vi "LoadCalcParPanel.vi"(4 "CalcProgQEvent":refnum<user-event>, 6 "CalcProgQ":refnum<queue>, 8 "error in (no error)":errorcluster caption="entrée d'erreur (pas d'erreur)", 9 "Session":i32, 11 "RemPanRef":refnum<vi>) -> (0 "sortie d'erreur":errorcluster, 2 "InstrClassEventQ":T1(array[cluster]), 3 "PanelViRefOut":refnum<vi>[](array[refnum]))   [LabVIEW 2019]
uses:
  Calculations Class/Calculations.lvclass
  C:/Programmes Labview/LabScanV1A/DevicesClass/BaseDevice/BaseDevice.lvclass
  DevicesClass/BaseDevice/BaseDevice.lvclass
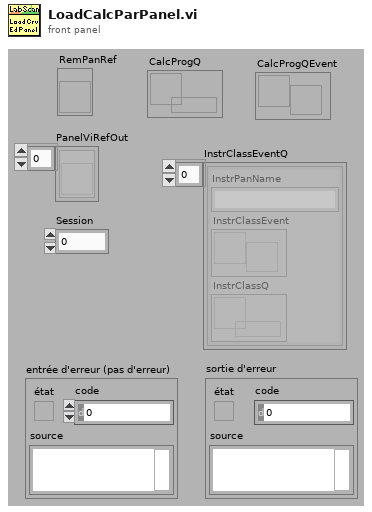
[diagram p1: front panel]
types:
  T1 = cluster{"InstrPanName":string, "InstrClassEvent":refnum<user-event>, "InstrClassQ":refnum<queue>}[]
  T2 = enum16{"Répertoire du VI actuel", "Répertoire du parent 1", "Répertoire du parent 2", "Répertoire du parent 3"}
  T3 = cluster{"Valeur":string, "InstrClassEvent":refnum<user-event>, "InstrClassQ":refnum<queue>}
  T4 = typedef "LVPointTypeDef.ctl" = cluster{"Horizontal":i16, "Vertical":i16}
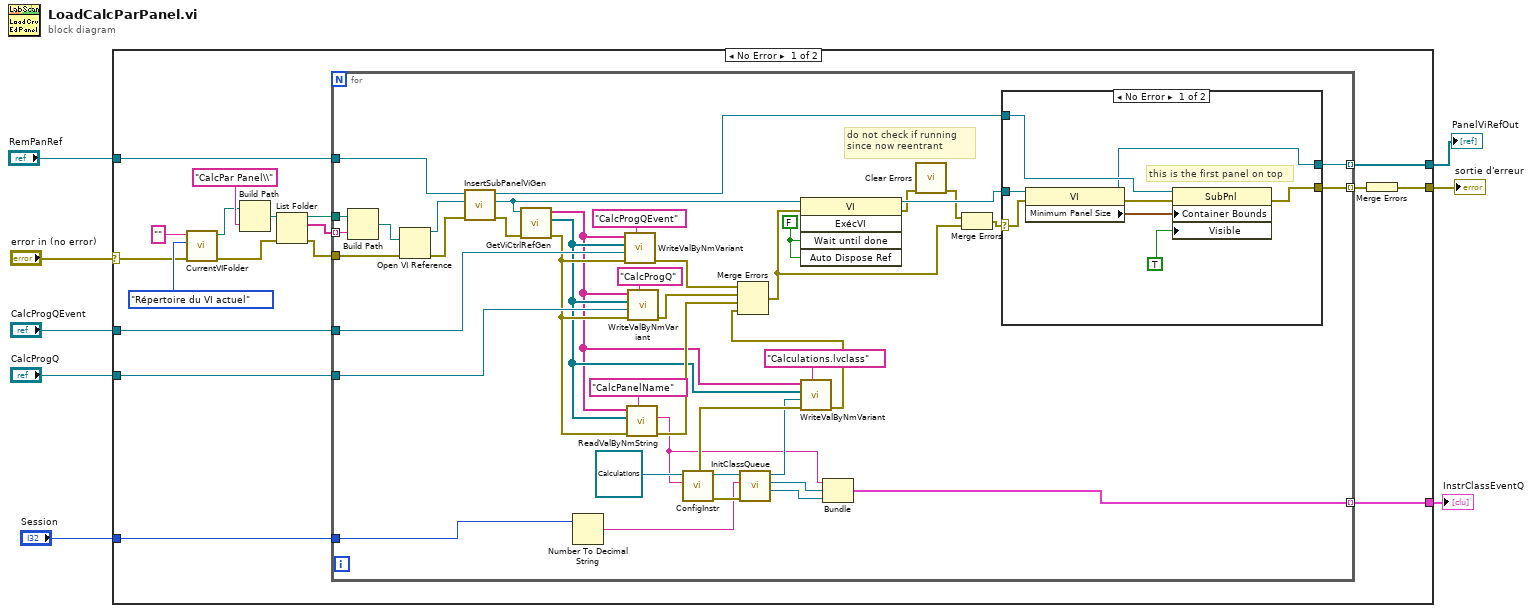
[diagram p0: block diagram]
diagram:
  n1 = case shown="No Error" "error in (no error)" {
    selector: "error in (no error)" -> [w13 w79]
    tunnel: [w26 w79] -> w7
    tunnel: "CalcProgQEvent" -> [w25 _]
    tunnel: "CalcProgQ" -> [w24 _]
    tunnel: "RemPanRef" -> [w22 _]
    tunnel: [w11 _] -> w3
    tunnel: "Session" -> [w10 _]
    tunnel: [w9 _] -> w1
    frame No Error {
      n2 = call <userlib>:"CurrentVIFolder.vi"("error in (no error)"=w13, "Source"=T2."Répertoire du VI actuel", "NomFichier"="") -> ("error out"=w19:errorcluster, "Chemin"=w16:path)  [unwired: 6 in, 1 out]
      n3 = Build Path(base path=w16, name or relative path="CalcPar Panel\\" ("nom ou chemin relatif")) -> (appended path=w18:path)
      n4 = List Folder(path=w18, error in=w19) -> (path out=w15:path, filenames=w14:string[], error out=w12:errorcluster)  [unwired: 2 in, 1 out]
      n5 = for {
        tunnel: w12 -> [w46]
        tunnel: [w66] -> w23 mode=indexing
        tunnel: w25 -> [w58]
        tunnel: w24 -> [w57]
        tunnel: w22 -> [w48]
        tunnel: w15 -> [w65]
        tunnel: w14 -> [w64] mode=indexing
        tunnel: [w62] -> w11 mode=indexing
        tunnel: w10 -> [w29]
        tunnel: [w30] -> w9 mode=indexing
        w67 = FALSE ("Attendre la fin")
        # "do not check if running \nsince now reentrant"
        n6 = Build Path(base path=w65, name or relative path=w64) -> (appended path=w63:path)
        n7 = Open VI Reference(vi path=w63, error in (no error)=w46) -> (vi reference=w44:refnum<vi>, error out=w45:errorcluster)  [unwired: 4 in]
        n8 = call <userlib>:"InsertSubPanelViGen.vi"("error in (no error)"=w45, "RemVIRef"=w44, "RemPanRef"=w48) -> ("sortie d'erreur"=w42:errorcluster, "RemVIRefOut"=w43:refnum<vi>, "RemPanRefOut"=w47:refnum<vi>)  [unwired: 6 in]
        n9 = call <userlib>:"GetViCtrlRefGen.vi"("ErrorIn(No Error)"=w42, "VIRef"=w43) -> ("sortie d'erreur"=w53:errorcluster, "ControlsRefs"=w36:refnum<vi>[], "ControlsNames"=w33:string[])  [unwired: 7 in]
        n10 = Number To Decimal String(number=w29) -> (decimal integer string=w38:string)  [unwired: 1 in]
        n11 = call <userlib>:"WriteValByNmVariant.vi"("Ctrl Name"="CalcProgQEvent" ("élément"), "error in"=w53, "Valeur"=w58, "CtrlRef"=w36, "ControlsNames"=w33) -> ("error out"=w51:errorcluster)  [unwired: 5 in, 1 out]
        n12 = call <userlib>:"ReadValByNmString.vi"("Ctrl Name"="CalcPanelName" ("élément"), "error in"=w53, "CtrlRef"=w36, "ControlsNames"=w33) -> ("error out"=w49:errorcluster, "Valeur"=w27:string)  [unwired: 5 in, 1 out]
        n13 = call <userlib>:"WriteValByNmVariant.vi"("Ctrl Name"="CalcProgQ" ("élément"), "error in"=w53, "Valeur"=w57, "CtrlRef"=w36, "ControlsNames"=w33) -> ("error out"=w50:errorcluster)  [unwired: 5 in, 1 out]
        n14 = call-dynamic "ConfigInstr.vi"("Function"=w27, "GenData In"=refnum<class "Calculations.lvclass"> refnum ("Calculations.lvclass")) -> ("error out"=w40:errorcluster, "GenData Out"=w39:refnum<class "Calculations.lvclass">)  [unwired: 8 in]
        n15 = call "InitClassQueue.vi"("ErrorIn(No Error)"=w40, "Session"=w38, "BaseDevice.lvclass"=w39) -> ("sortie d'erreur"=w37:errorcluster, "InstrClassQ"=w31:refnum<queue>, "InstrClassEvent"=w28:refnum<user-event>, "BaseDevice.lvclass Out"=w34:refnum<class "Calculations.lvclass">)  [unwired: 5 in]
        n16 = call <userlib>:"WriteValByNmVariant.vi"("Ctrl Name"="Calculations.lvclass", "error in"=w37, "Valeur"=w34, "CtrlRef"=w36, "ControlsNames"=w33) -> ("error out"=w32:errorcluster)  [unwired: 5 in, 1 out]
        n17 = Merge Errors(w51, w50, w49, w32) -> (w52:errorcluster)
        n18 = invoke class="VI" method="ExécVI"(reference=w43, error in=w52, "Wait until done"=w67, "Auto Dispose Ref"=w67) -> (reference out=w68:refnum<vi>, error out=w60:errorcluster)  [unwired: 1 in, 3 out]
        n19 = Bundle("Valeur"=w27, "InstrClassEvent"=w28, "InstrClassQ"=w31) -> (w30:T3)  [unwired: 1 in]
        n20 = call <vilib>:"Clear Errors.vi"("error in (no error)"=w60) -> ("error out"=w59:errorcluster)  [unwired: 5 in, 1 out]
        n21 = Merge Errors(w59, w52) -> (w61:errorcluster)
        n22 = case shown="No Error" w61 {
          selector: w61 -> [w73 w78]
          tunnel: [w71 w78] -> w66
          tunnel: w47 -> [w74 _]
          tunnel: w68 -> [w72 w77]
          tunnel: [w69 w77] -> w62
          frame No Error {
            # "this is the first panel on top"
            n23 = property class="VI"(reference=w72, error in=w73) -> (reference out=w69:refnum<vi>, error out=w75:errorcluster, "Minimum Panel Size"=w76:T4)
            n24 = property class="SubPnl"(reference=w74, error in=w75, "Container Bounds"=w76, "Visible"=TRUE) -> (error out=w71:errorcluster)  [unwired: 1 out]
          }
          frame Error {
          }
        }
      }
      n25 = Merge Errors(w23) -> (w26:errorcluster)
    }
    frame Error {
    }
  }
  "sortie d'erreur" <- w7
  "PanelViRefOut" <- w3
  "InstrClassEventQ" <- w1
